vi "PS Class Load.vi"(8 "error in (no error)":errorcluster, 9 "PS Type":T1, 11 "PS in":refnum<class "PS.lvclass">) -> (0 "error out":errorcluster, 3 "PS out":refnum<class "PS.lvclass">)   [LabVIEW 2021, in "PS.lvlib"]
doc: "<b>Note:</b> This VI was modified by the <b>Validate DQMH Module</b> tool to turn off automatic error handling."
uses:
  PS.lvlib
  td_en_pstype.ctl
  Custom/PS/PS.lvclass
  Custom/PS Keysight/PS Keysight.lvclass
  Custom/PS Simulated/PS Simulated.lvclass
  Custom/PS Test/PS Test.lvclass
  C:/Projects/lbaute/InstrPanel/Libraries/PS/Custom/PS/PS.lvclass
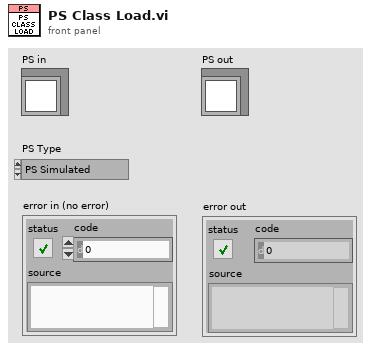
[diagram p1: front panel]
types:
  T1 = typedef "PS.lvlib/td_en_pstype.ctl" = enum16{"PS Simulated", "Keysight E3642A", "PS Test", "PS"}
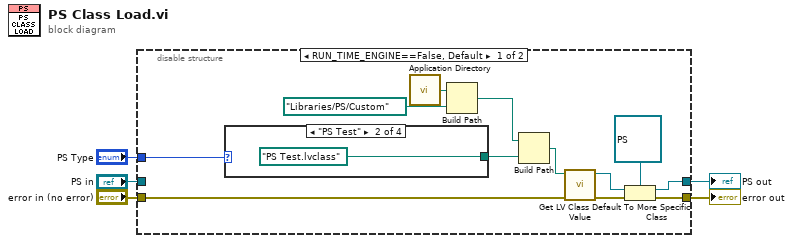
[diagram p0: block diagram]
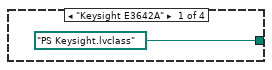
[diagram p2: hidden frame]
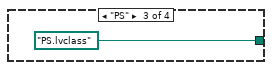
[diagram p3: hidden frame]
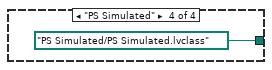
[diagram p4: hidden frame]
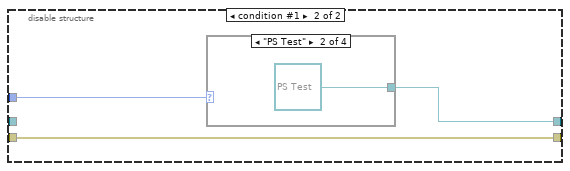
[diagram p5: hidden frame]
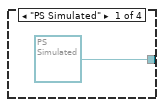
[diagram p6: hidden frame]
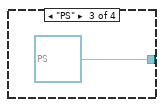
[diagram p7: hidden frame]
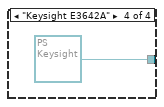
[diagram p8: hidden frame]
diagram:
  n1 = disable-structure shown="RUN_TIME_ENGINE==False, Default" {
    disable-tunnel: "PS Type" -> [w17 w23]
    disable-tunnel: [w13 w22] -> w2
    disable-tunnel: [w11 w24] -> w4
    disable-tunnel: "error in (no error)" -> [w9 w24]
    disable-tunnel: "PS in" -> [_ _]
    frame condition #0 (active) {
      n2 = case shown="\"PS Test\"" w17 {
        tunnel: [path "PS Keysight.lvclass" path "PS Test.lvclass" path "PS.lvclass" path "PS Simulated/PS Simulated.lvclass"] -> w16
        frame "Keysight E3642A" {
        }
        frame "PS Test" {
        }
        frame "PS" {
        }
        frame "PS Simulated" {
        }
      }
      n3 = call <vilib>:"Application Directory.vi"() -> ("Application Directory"=w8:path)
      n4 = Build Path(base path=w8, name or relative path=path "Libraries/PS/Custom" ("Classes Directory")) -> (appended path=w6:path)
      n5 = Build Path(base path=w6, name or relative path=w16) -> (appended path=w15:path)
      n6 = call <vilib>:"Get LV Class Default Value.vi"("error in (no error)"=w9, "class path"=w15) -> ("error out"=w10:errorcluster, "object"=w14:refnum<class>)  [unwired: 8 in]
      n7 = To More Specific Class(target class=refnum<class "PS.lvclass"> refnum ("PS.lvclass"), reference=w14, error in=w10) -> (specific class reference=w13:refnum<class "PS.lvclass">, error out=w11:errorcluster)
    }
    frame condition #1 {
      n8 = case shown="\"PS Test\"" w23 {
        tunnel: [refnum<class "PS Simulated.lvclass"> refnum ("PS:PS Sim") refnum<class "PS Test.lvclass"> refnum ("PS:PS Test.lvclass") refnum<class "PS.lvclass"> refnum ("PS:PS.lvclass") refnum<class "PS Keysight.lvclass"> refnum ("PS:Keysight")] -> w22
        frame "PS Simulated" {
        }
        frame "PS Test" {
        }
        frame "PS" {
        }
        frame "Keysight E3642A" {
        }
      }
    }
  }
  "PS out" <- w2
  "error out" <- w4
